vi "FGV_VI-REF.vi"(8 "error in (no error)":errorcluster caption="entrée d'erreur (pas d'erreur)", 10 "Data_IN":refnum<vi>, 11 "Action":T1=enum."GET") -> (0 "error out":errorcluster caption="sortie d'erreur", 2 "Data_OUT":refnum<vi>)   [LabVIEW 2013]
uses:
  Action.ctl
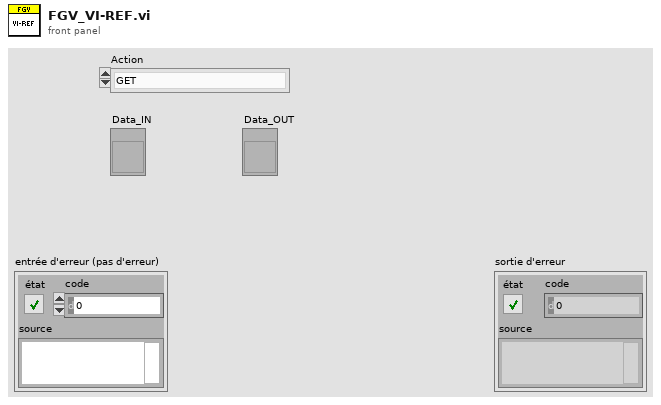
[diagram p1: front panel]
types:
  T1 = typedef "Action.ctl" = enum16{"SET", "GET"}
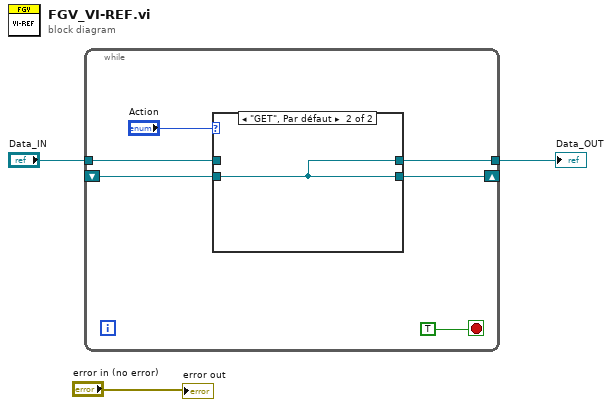
[diagram p0: block diagram]
diagram:
  n1 = while {
    shift-right: [w8] -> _
    shift-left: _ -> [w6]
    tunnel: "Data_IN" -> [w9]
    tunnel: [w7] -> w2
    stop <- TRUE stop-if-true
    n2 = case shown="\"GET\", Par défaut" "Action" {
      tunnel: w9 -> [w10 _]
      tunnel: [w10 w11] -> w8
      tunnel: [w10 w11] -> w7
      tunnel: w6 -> [_ w11]
      frame "SET" {
      }
      frame "GET", Default {
      }
    }
  }
  "Data_OUT" <- w2
  "error out" <- "error in (no error)"
